vi "read TBM configuration.vi"(8 "error in":errorcluster, 11 "Standard Engine Editor Node in":refnum<class "Standard Engine Editor Node.lvclass">) -> (0 "error out":errorcluster, 2 "configuration":refnum<class "TBM configuration.lvclass">, 3 "Standard Engine Editor Node out":refnum<class "Standard Engine Editor Node.lvclass">)   [LabVIEW 2013, in "Standard Engine Editor Node.lvclass"]
uses:
  Standard Engine Editor Node.lvclass
  <vilib>/NI/Tag Bus Module Framework/root configuration/TBM configuration.lvclass
  Standard Engine Editor Node.lvclass/Standard Engine Editor Node.ctl
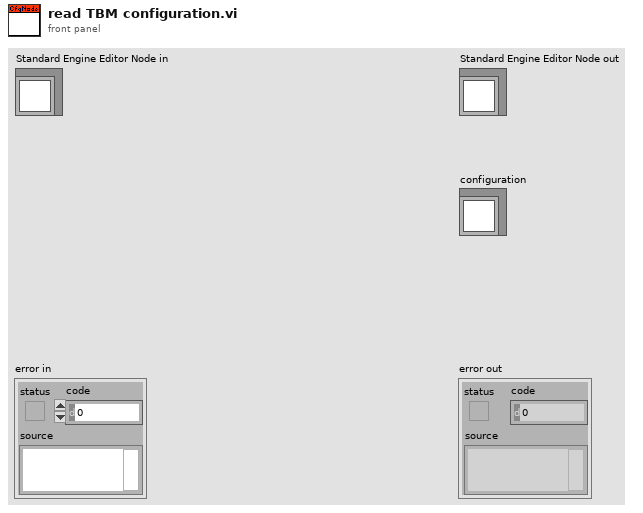
[diagram p1: front panel]
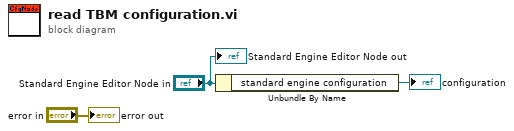
[diagram p0: block diagram]
diagram:
  n1 = Unbundle By Name("Standard Engine Editor Node in") -> ("standard engine configuration"=→"configuration":refnum<class "Standard Engine Configuration.lvclass">)
  "error out" <- "error in"
  "Standard Engine Editor Node out" <- "Standard Engine Editor Node in"
